vi "task 2a.vi"() -> ()   [LabVIEW 2017]
uses:
  <vilib>/DAQmx/read.llb/DAQmx Read (Digital Bool 1Line 1Point).vi
  <vilib>/DAQmx/write.llb/DAQmx Write (Analog DBL 1Chan 1Samp).vi
  <vilib>/DAQmx/create/channels.llb/DAQmx Create Channel (AO-Voltage-Basic).vi
  <vilib>/DAQmx/create/channels.llb/DAQmx Create Channel (DI-Digital Input).vi
  <vilib>/DAQmx/miscellaneous.llb/DAQmx Fill In Error Info.vi
panel:
  out "Right":bool
  out "Bottom":bool
  out "Left":bool
  out "Top":bool
  in  "DAQmx Physical Channel 6":tag
  in  "DAQmx Physical Channel 5":tag
  in  "DAQmx Physical Channel 4":tag
  in  "DAQmx Physical Channel 3":tag
  in  "Motor stop":bool
  in  "DAQmx Physical Channel 2":tag="Dev9/ao0"
  in  "motor 2":dbl(slide)=3.2073478842720426 scale=0.0..10.0
  in  "max Voltage":dbl
  in  "Min Voltage":dbl
  in  "DAQmx Physical Channel":tag="Dev9/ao0"
  in  "motor 1":dbl(slide)=3.2073478842720426 scale=0.0..10.0
  in  "stop":bool
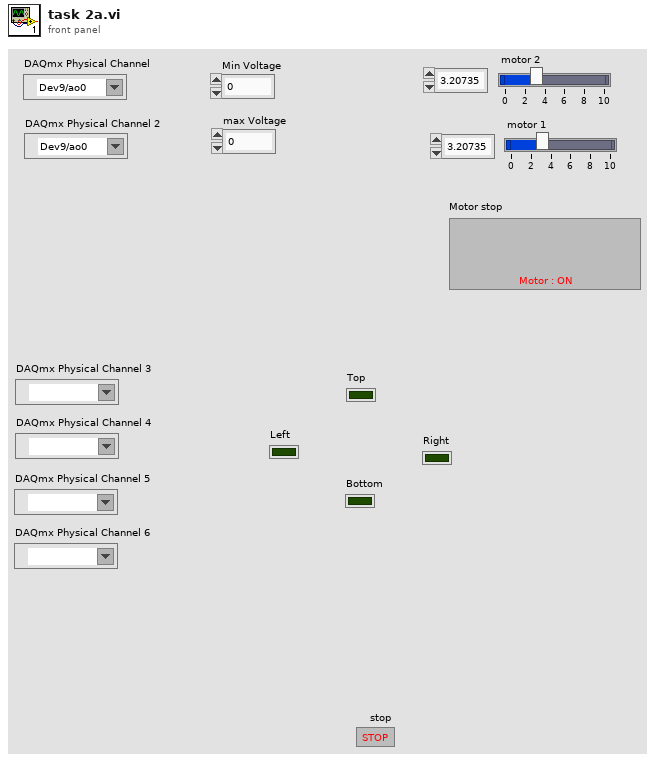
[diagram p1: front panel]
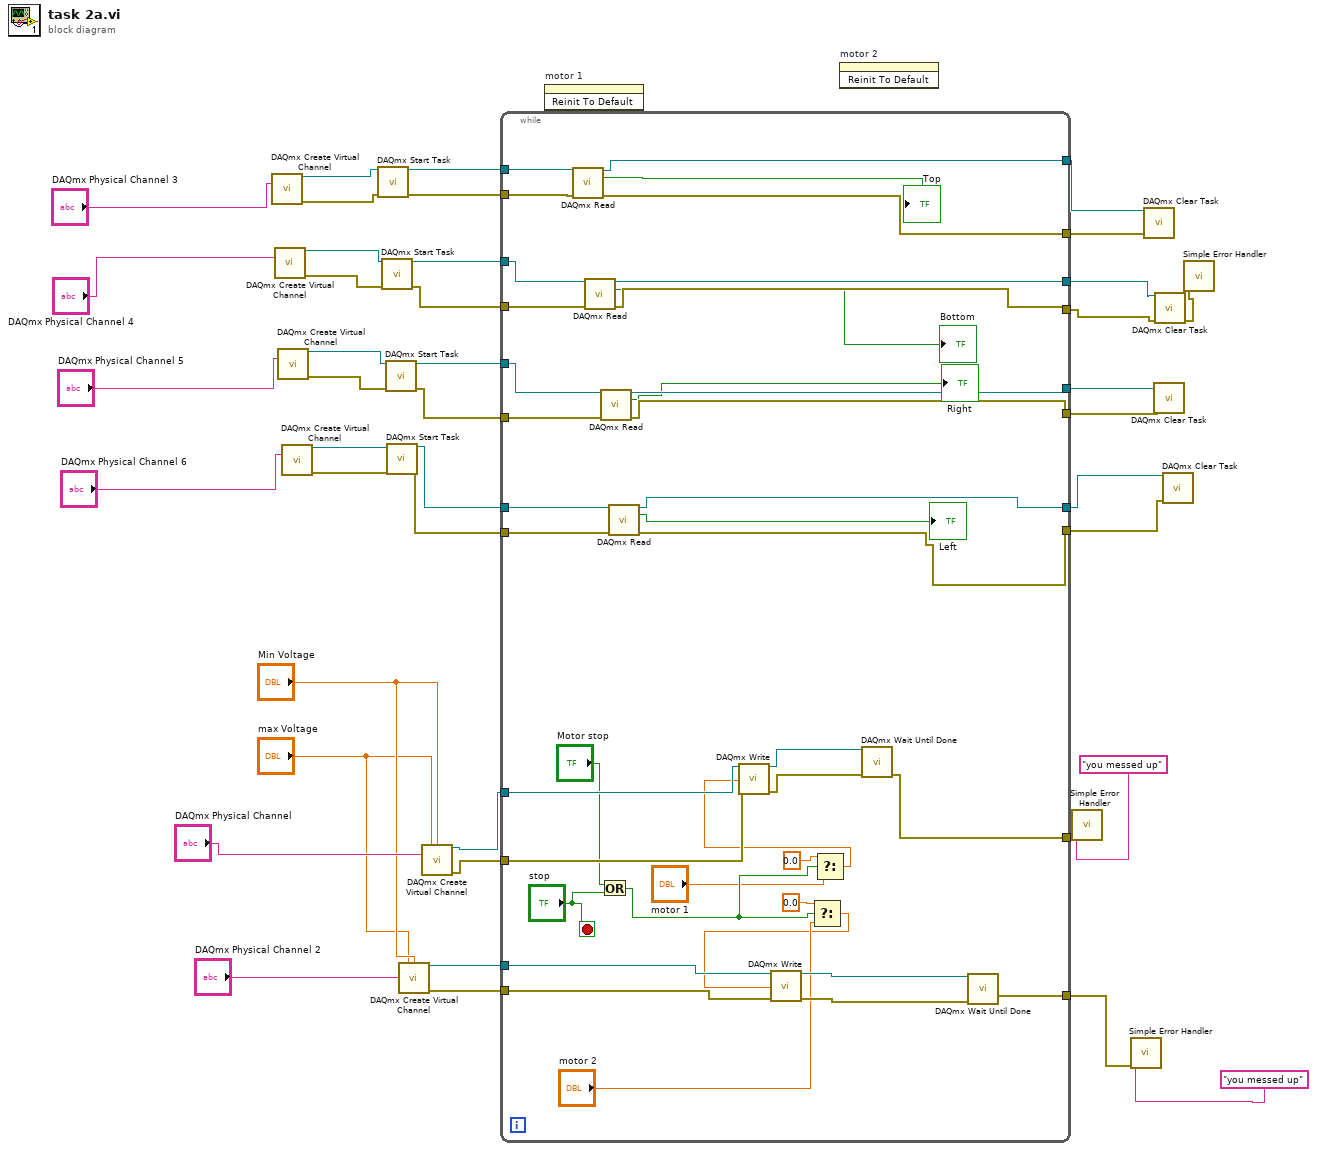
[diagram p0: block diagram]
diagram:
  n1 = call-poly <vilib>:"DAQmx Create Virtual Channel.vi"("lines"="DAQmx Physical Channel 3") -> ("task out"=w25:refnum<k21>, "error out"=w21:errorcluster)  [unwired: 13 in]
  n2 = call-poly <vilib>:"DAQmx Create Virtual Channel.vi"("lines"="DAQmx Physical Channel 4") -> ("task out"=w24:refnum<k21>, "error out"=w20:errorcluster)  [unwired: 13 in]
  n3 = call-poly <vilib>:"DAQmx Create Virtual Channel.vi"("lines"="DAQmx Physical Channel 5") -> ("task out"=w23:refnum<k21>, "error out"=w19:errorcluster)  [unwired: 13 in]
  n4 = call-poly <vilib>:"DAQmx Create Virtual Channel.vi"("lines"="DAQmx Physical Channel 6") -> ("task out"=w22:refnum<k21>, "error out"=w18:errorcluster)  [unwired: 13 in]
  n5 = call <vilib>:"DAQmx Start Task.vi"("task/channels in"=w25, "error in"=w21) -> ("task out"=w17:refnum<k21>, "error out"=w15:errorcluster)  [unwired: 12 in]
  n6 = call <vilib>:"DAQmx Start Task.vi"("task/channels in"=w24, "error in"=w20) -> ("task out"=w13:refnum<k21>, "error out"=w10:errorcluster)  [unwired: 12 in]
  n7 = call <vilib>:"DAQmx Start Task.vi"("task/channels in"=w23, "error in"=w19) -> ("task out"=w12:refnum<k21>, "error out"=w9:errorcluster)  [unwired: 12 in]
  n8 = call <vilib>:"DAQmx Start Task.vi"("task/channels in"=w22, "error in"=w18) -> ("task out"=w11:refnum<k21>, "error out"=w8:errorcluster)  [unwired: 12 in]
  n9 = call-poly <vilib>:"DAQmx Create Virtual Channel.vi"("maximum value"="max Voltage", "minimum value"="Min Voltage", "physical channels"="DAQmx Physical Channel 2") -> ("task out"=w35:refnum<k21>, "error out"=w31:errorcluster)  [unwired: 11 in]
  n10 = call-poly <vilib>:"DAQmx Create Virtual Channel.vi"("maximum value"="max Voltage", "minimum value"="Min Voltage", "physical channels"="DAQmx Physical Channel") -> ("task out"=w39:refnum<k21>, "error out"=w30:errorcluster)  [unwired: 11 in]
  n11 = while {
    tunnel: w39 -> [w80]
    tunnel: [w77] -> w38
    tunnel: w35 -> [w74]
    tunnel: [w73] -> w34
    tunnel: w31 -> [w71]
    tunnel: w30 -> [w70]
    tunnel: w17 -> [w61]
    tunnel: [w60] -> w16
    tunnel: w15 -> [w59]
    tunnel: [w58] -> w14
    tunnel: w13 -> [w57]
    tunnel: w12 -> [w56]
    tunnel: w11 -> [w55]
    tunnel: w10 -> [w54]
    tunnel: w9 -> [w53]
    tunnel: w8 -> [w52]
    tunnel: [w51] -> w7
    tunnel: [w50] -> w6
    tunnel: [w49] -> w5
    tunnel: [w48] -> w4
    tunnel: [w47] -> w3
    tunnel: [w46] -> w2
    stop <- "stop" stop-if-true
    n12 = call-poly <vilib>:"DAQmx Read.vi"("task/channels in"=w61, "error in"=w59) -> ("task out"=w60:refnum<k21>, "data"=→"Top":bool, "error out"=w58:errorcluster)  [unwired: 11 in]
    n13 = call-poly <vilib>:"DAQmx Read.vi"("task/channels in"=w57, "error in"=w54) -> ("task out"=w51:refnum<k21>, "data"=→"Bottom":bool, "error out"=w48:errorcluster)  [unwired: 11 in]
    n14 = Or(x="Motor stop", y="stop") -> (x .or. y?=w66:bool)
    n15 = call-poly <vilib>:"DAQmx Read.vi"("task/channels in"=w56, "error in"=w53) -> ("task out"=w50:refnum<k21>, "data"=→"Right":bool, "error out"=w47:errorcluster)  [unwired: 11 in]
    n16 = call-poly <vilib>:"DAQmx Read.vi"("task/channels in"=w55, "error in"=w52) -> ("task out"=w49:refnum<k21>, "data"=→"Left":bool, "error out"=w46:errorcluster)  [unwired: 11 in]
    n17 = Select(t=0.0, s=w66, f="motor 2") -> (s? t:f=w62:dbl)
    n18 = call-poly <vilib>:"DAQmx Write.vi"("task/channels in"=w74, "data"=w62, "error in"=w71) -> ("task out"=w75:refnum<k21>, "error out"=w76:errorcluster)  [unwired: 10 in, 1 out]
    n19 = Select(t=0.0 ("s? t:f"), s=w66, f="motor 1") -> (s? t:f=w63:dbl)
    n20 = call-poly <vilib>:"DAQmx Write.vi"("task/channels in"=w80, "data"=w63, "error in"=w70) -> ("task out"=w79:refnum<k21>, "error out"=w78:errorcluster)  [unwired: 10 in, 1 out]
    n21 = call <vilib>:"DAQmx Wait Until Done.vi"("task/channels in"=w79, "error in"=w78) -> ("error out"=w77:errorcluster)  [unwired: 12 in, 1 out]
    n22 = call <vilib>:"DAQmx Wait Until Done.vi"("task/channels in"=w75, "error in"=w76) -> ("error out"=w73:errorcluster)  [unwired: 12 in, 1 out]
  }
  n23 = invoke on="motor 1" class="Slide (strict)" method="Reinit To Default"() -> ()  [unwired: 3 in, 3 out]
  n24 = invoke on="motor 2" class="Slide (strict)" method="Reinit To Default"() -> ()  [unwired: 3 in, 3 out]
  n25 = call <vilib>:"Simple Error Handler.vi"("error source (\" \")"="you messed up" ("error source (\" \")"), "error in (no error)"=w38) -> ()  [unwired: 3 in, 5 out]
  n26 = call <vilib>:"Simple Error Handler.vi"("error source (\" \")"="you messed up" ("error source (\" \")"), "error in (no error)"=w34) -> ()  [unwired: 3 in, 5 out]
  n27 = call <vilib>:"DAQmx Clear Task.vi"("task in"=w16, "error in"=w14) -> ()  [unwired: 13 in, 1 out]
  n28 = call <vilib>:"DAQmx Clear Task.vi"("task in"=w6, "error in"=w3) -> ()  [unwired: 13 in, 1 out]
  n29 = call <vilib>:"DAQmx Clear Task.vi"("task in"=w7, "error in"=w4) -> ("error out"=w1:errorcluster)  [unwired: 13 in]
  n30 = call <vilib>:"DAQmx Clear Task.vi"("task in"=w5, "error in"=w2) -> ()  [unwired: 13 in, 1 out]
  n31 = call <vilib>:"Simple Error Handler.vi"("error in (no error)"=w1) -> ()  [unwired: 4 in, 5 out]
